vi "Close.vi"(8 "error in (no error)":errorcluster) -> (0 "error out":errorcluster)   [LabVIEW 2018, in "Receipt Parsing.lvlib"]
uses:
  Receipt Parsing.lvlib
  Action.ctl
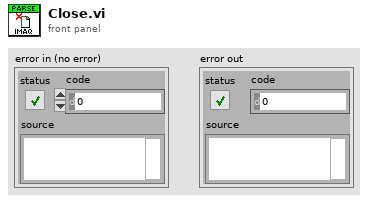
[diagram p1: front panel]
types:
  T1 = typedef "Receipt Parsing.lvlib/Action.ctl" = enum16{"Init", "Read Image Text", "Close"}
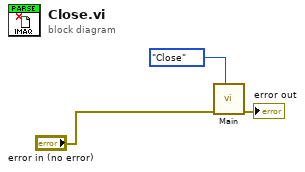
[diagram p0: block diagram]
diagram:
  n1 = call "Main.vi"("Action"=Action."Close", "Error In"="error in (no error)") -> ("Error Out"=→"error out":errorcluster)  [unwired: 8 in, 1 out]
